vi "Method 2.vi"(8 "error in (no error)":errorcluster, 11 "Child in":refnum<class "Child.lvclass">) -> (0 "error out":errorcluster, 3 "Child out":refnum<class "Child.lvclass">)   [LabVIEW 2021, in "Child.lvclass"]
uses:
  Child.lvclass
  Child.lvclass/Child.ctl
  Interface/Interface.lvclass
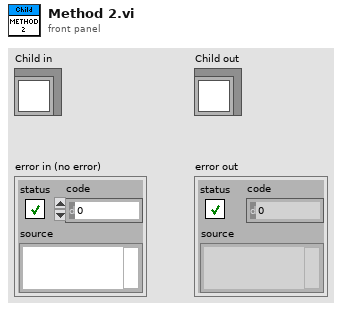
[diagram p1: front panel]
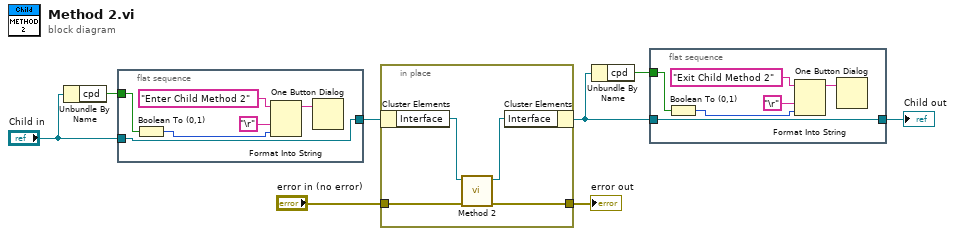
[diagram p0: block diagram]
diagram:
  n1 = Unbundle By Name("Child in") -> ("cpd"=w2:bool)
  n2 = flat-sequence {
    tunnel: [w14] -> w6
    tunnel: "Child in" -> [w14]
    tunnel: w2 -> [w13]
    frame #0 {
      n3 = Boolean To (0,1)(Boolean=w13) -> (0, 1=w10:i16)
      n4 = Format Into String(initial string="Enter Child Method 2" ("message"), "\r", w10) -> (resulting string=w12:string)  [unwired: 2 in, 1 out]
      n5 = One Button Dialog(message=w12) -> ()  [unwired: 1 in, 1 out]
    }
  }
  n6 = in-place {
    in-place-border: "error in (no error)" -> [w16]
    in-place-border: [w15] -> w7
    n7 = in-place-cluster #1(w6) -> ("Interface"=w18:refnum<class "Interface.lvclass">)
    n8 = call-dynamic "Method 2.vi"("error in (no error)"=w16, "Interface 2 in"=w18) -> ("error out"=w15:errorcluster, "Interface 2 out"=w17:refnum<class "Interface.lvclass">)  [unwired: 8 in]
    n9 = in-place-cluster #1("Interface"=w17) -> (w3:refnum<class "Child.lvclass">)
  }
  "error out" <- w7
  n10 = Unbundle By Name(w3) -> ("cpd"=w1:bool)
  n11 = flat-sequence {
    tunnel: [w24] -> w5
    tunnel: w3 -> [w24]
    tunnel: w1 -> [w21]
    frame #0 {
      n12 = Boolean To (0,1)(Boolean=w21) -> (0, 1=w23:i16)
      n13 = Format Into String(initial string="Exit Child Method 2" ("message"), "\r", w23) -> (resulting string=w19:string)  [unwired: 2 in, 1 out]
      n14 = One Button Dialog(message=w19) -> ()  [unwired: 1 in, 1 out]
    }
  }
  "Child out" <- w5
